vi "MPB Sequences.vi"(10 "sequence number":i32) -> (2 "(description) used in test":string)   [LabVIEW 2020]
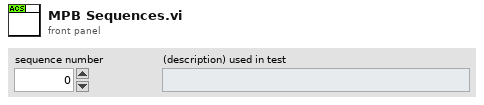
[diagram p1: front panel]
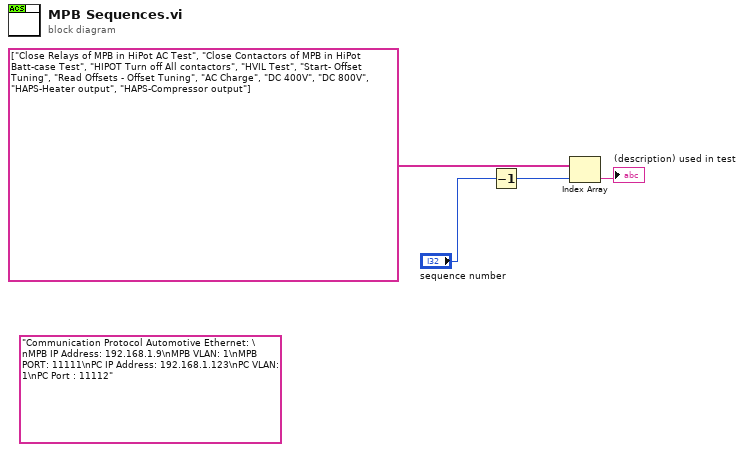
[diagram p0: block diagram]
diagram:
  (unwired) "Communication Protocol Automotive Ethernet: \nMPB IP Address: 192.168.1.9\nMPB VLAN: 1\nMPB PORT: 11111\nPC IP Address: 192.168.1.123\nPC VLAN: 1\nPC Port : 11112"
  n1 = Decrement(x="sequence number") -> (x-1=w2:i32)
  n2 = Index Array(array=string[] ["Close Relays of MPB in HiPot AC Test", "Close Contactors of MPB in HiPot Batt-case Test", "HIPOT Turn off All contactors", "HVIL Test", "Start- Offset Tuning", "Read Offsets - Offset Tuning", "AC Charge", "DC 400V", "DC 800V", "HAPS-Heater output", "HAPS-Compressor output"], index=w2) -> (element=→"(description) used in test":string)
